vi "Load Subpanel.vi"(8 "error in (no error)":errorcluster, 10 "Subpanel Type":T1, 11 "CIF_UI in":refnum<class "CIF_UI.lvclass">) -> (0 "error out":errorcluster, 2 "VI Reference":refnum<vi>, 3 "CIF_UI out":refnum<class "CIF_UI.lvclass">)   [LabVIEW 2021, in "CIF_UI.lvclass"]
uses:
  CIF_UI.lvclass
  Typedef/Subpanel Type.ctl
  CIF_UI.lvclass/CIF_UI.ctl
  Typedef/Subpanel Data.ctl
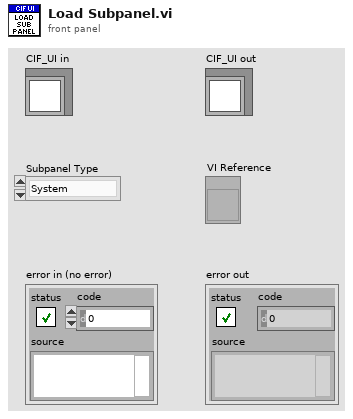
[diagram p1: front panel]
types:
  T1 = typedef "CIF_UI.lvclass/Subpanel Type.ctl" = enum16{"System", "Errors", "Channel", "Plugin"}
  T2 = typedef "CIF_UI.lvclass/Subpanel Data.ctl" = cluster{"VI Reference":refnum<vi>}
  T3 = typedef "CIF_UI.lvclass/Subpanel Map.ctl" = map{T1, T2}
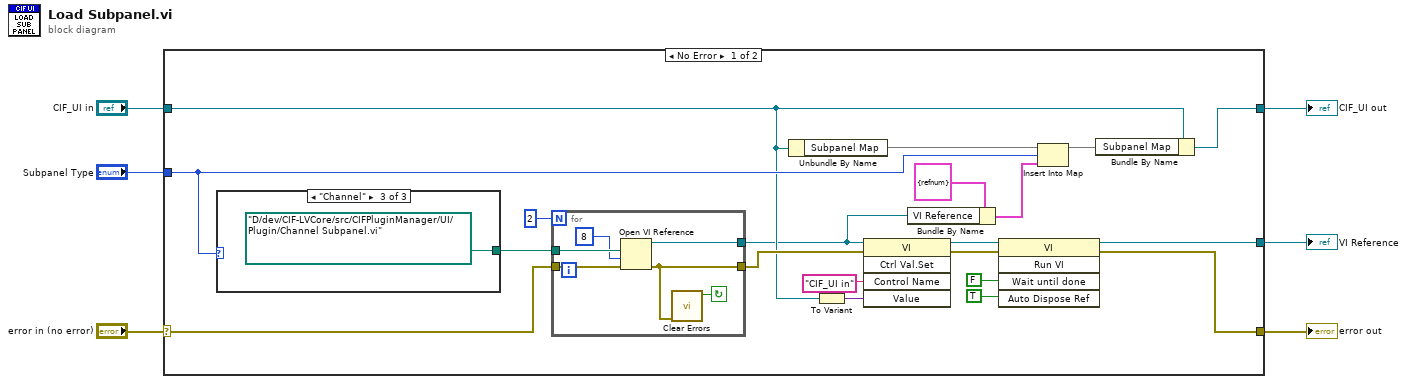
[diagram p0: block diagram]
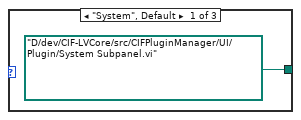
[diagram p2: hidden frame]
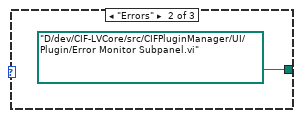
[diagram p3: hidden frame]
diagram:
  n1 = case shown="No Error" "error in (no error)" {
    selector: "error in (no error)" -> [w13 w37]
    tunnel: [w12 w37] -> w5
    tunnel: [w9 w36] -> w3
    tunnel: "CIF_UI in" -> [w11 w36]
    tunnel: "Subpanel Type" -> [w14 _]
    tunnel: [w8 _] -> w1
    frame No Error {
      n2 = case shown="\"Channel\"" w14 {
        tunnel: [path "D:/dev/CIF-LVCore/src/CIFPluginManager/UI/Plugin/System Subpanel.vi" ("Linux") path "D:/dev/CIF-LVCore/src/CIFPluginManager/UI/Plugin/Error Monitor Subpanel.vi" ("Linux") path "D:/dev/CIF-LVCore/src/CIFPluginManager/UI/Plugin/Channel Subpanel.vi" ("Linux")] -> w17
        frame "System", Default {
        }
        frame "Errors" {
        }
        frame "Channel" {
        }
      }
      n3 = for {
        N: 2 -> [_]
        tunnel: w17 -> [w35]
        tunnel: [w34] -> w7
        tunnel: [w32] -> w23
        tunnel: w13 -> [w30]
        stop <- w31 continue-if-true
        n4 = Open VI Reference(vi path=w35, options=8, error in (no error)=w30) -> (vi reference=w34:refnum<vi>, error out=w32:errorcluster)  [unwired: 3 in]
        n5 = call <vilib>:"Clear Errors.vi"("error in (no error)"=w32) -> ("specific error cleared?"=w31:bool)  [unwired: 5 in, 1 out]
      }
      n6 = Unbundle By Name(w11) -> ("Subpanel Map"=w16:T3)
      n7 = To Variant(anything=w11) -> (Variant=w19:variant)
      n8 = invoke class="VI" method="Ctrl Val.Set"(reference=w7, error in=w23, "Control Name"="CIF_UI in", "Value"=w19) -> (reference out=w24:refnum<vi>, error out=w25:errorcluster)  [unwired: 1 in, 3 out]
      n9 = Bundle By Name(cluster=T2 {"VI Reference"=refnum} ("SubPanel Data"), "VI Reference"=w7) -> (w15:T2)
      n10 = invoke class="VI" method="Run VI"(reference=w24, error in=w25, "Wait until done"=FALSE ("Wait Until Done"), "Auto Dispose Ref"=TRUE ("Auto Dispose Reference")) -> (reference out=w8:refnum<vi>, error out=w12:errorcluster)  [unwired: 1 in, 3 out]
      n11 = Insert Into Map(map in=w16, key=w14, value=w15) -> (map out=w10:T3)  [unwired: 2 out]
      n12 = Bundle By Name(cluster=w11, "Subpanel Map"=w10) -> (w9:refnum<class "CIF_UI.lvclass">)
    }
    frame Error {
    }
  }
  "error out" <- w5
  "CIF_UI out" <- w3
  "VI Reference" <- w1
